vi "_Prompt Tree.vi"   [LabVIEW 2011]
uses:
  LIB/Prompt Version.vi
panel:
  # "See Diagram"
types:
  T1 = typedef "OGAB Version.ctl" = cluster{"Version":string, "Build Number":u32, "Build Date/Time":dbl}
  T2 = typedef "Field Record.ctl" = cluster{"ixField":i32, "iSequenceOrder":i32, "sxFieldId":string, "sxSequenceId":string, "sDisplayName":string, "sValue":string, "sUnits":string, "nDataType":T3, "nNextItem":T4, "fSystem":bool, "fSystemValue":bool, "fRequired":bool, "fSetAtTest":bool, "fTestField":bool, "fDeleted":bool, "fIndexed":bool, "fFreeList":bool}
  T3 = typedef "Field DataTypes.ctl" = enum32{"text", "numeric", "list", "timestamp", "boolean"}
  T4 = typedef "Field NextItem.ctl" = enum32{"Reset", "Retain", "Auto-Increment"}
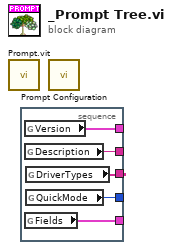
[diagram p0: block diagram]
diagram:
  n1 = call "Prompt.vit"() -> ()  [unwired: 4 in, 8 out]
  n2 = stacked-sequence {
    tunnel: [w5] -> _
    tunnel: [w4] -> _
    tunnel: [w3] -> _
    tunnel: [w2] -> _
    tunnel: [w1] -> _
    frame #0 {
      n3 = global read "Prompt Version.vi" "Version"() -> (w2:T1)
      n4 = global read "Prompt Version.vi" "Description"() -> (w3:string)
      n5 = global read "Prompt Version.vi" "Fields"() -> (w1:T2[])
      n6 = global read "Prompt Version.vi" "DriverTypes"() -> (w4:string[])
      n7 = global read "Prompt Version.vi" "QuickMode"() -> (w5:i32)
    }
  }
  n8 = call "Prompt Configuration.vi"() -> ()  [unwired: 5 in, 7 out]
